vi "enviarMensagem.vi"(8 "error in (no error)":errorcluster, 11 "Cliente in":refnum<class "Cliente.lvclass">) -> (0 "error out":errorcluster, 2 "ok":bool, 3 "Cliente out":refnum<class "Cliente.lvclass">, 4 "msg_recebida":string, 6 "msg_enviada":string)   [LabVIEW 2016, in "Cliente.lvclass"]
uses:
  Cliente.lvclass
  Cliente.lvclass/Cliente.ctl
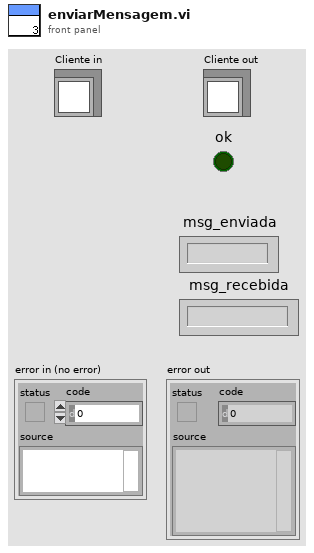
[diagram p1: front panel]
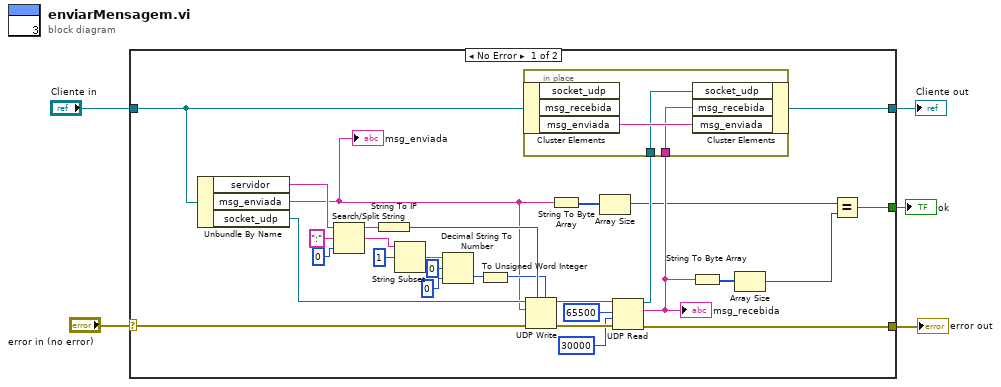
[diagram p0: block diagram]
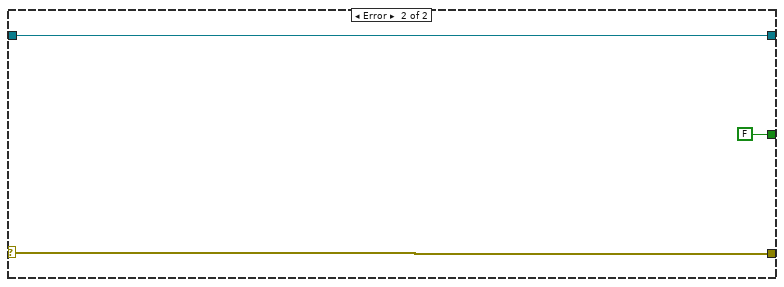
[diagram p2: hidden frame]
diagram:
  n1 = case shown="No Error" "error in (no error)" {
    selector: "error in (no error)" -> [w19 w40]
    tunnel: [w20 w40] -> w5
    tunnel: [w34 w38] -> w4
    tunnel: [w14 FALSE] -> w3
    tunnel: "Cliente in" -> [w15 w38]
    frame No Error {
      n2 = Unbundle By Name(w15) -> ("servidor"=w16:string, "msg_enviada"=w11:string, "socket_udp"=w17:refnum<k16>)
      "msg_enviada" <- w11
      n3 = Search/Split String(string=w16, search string/char (-)=":", offset (0)=0) -> (substring before match=w29:string, match + rest of string=w26:string)  [unwired: 1 out]
      n4 = String To IP(1:w29) -> (0:w28:u32)
      n5 = String Subset(string=w26, offset (0)=1) -> (substring=w25:string)  [unwired: 1 in]
      n6 = Decimal String To Number(string=w25, offset=0, default (0L)=0 ("default (0 I32)")) -> (number=w21:i32)  [unwired: 1 out]
      n7 = To Unsigned Word Integer(number=w21) -> (unsigned 16bit integer=w22:u16)
      n8 = UDP Write(address=w28, port or service name=w22, connection ID=w17, data in=w11, 8:w19) -> (error out=w32:errorcluster, 3:w33:refnum<k16>)  [unwired: 1 in]
      n9 = String To Byte Array(string=w11) -> (unsigned byte array=w10:u8[])
      n10 = Array Size(array=w10) -> (size(s)=w7:i32)
      n11 = UDP Read(connection ID=w33, max size (548)=65500, timeout ms (25000)=30000, 8:w32) -> (data out=w12:string, error out=w20:errorcluster, 3:w18:refnum<k16>)  [unwired: 2 out]
      "msg_recebida" <- w12
      n12 = in-place {
        in-place-border: w18 -> [w36]
        in-place-border: w12 -> [w35]
        n13 = in-place-cluster #1(w15) -> ("msg_enviada"=w37:string)  [unwired: 2 out]
        n14 = in-place-cluster #1("socket_udp"=w36, "msg_recebida"=w35, "msg_enviada"=w37) -> (w34:refnum<class "Cliente.lvclass">)
      }
      n15 = String To Byte Array(string=w12) -> (unsigned byte array=w9:u8[])
      n16 = Array Size(array=w9) -> (size(s)=w8:i32)
      n17 = Equal?(x=w7, y=w8) -> (x = y?=w14:bool)
    }
    frame Error {
    }
  }
  "error out" <- w5
  "Cliente out" <- w4
  "ok" <- w3
